vi "item select new.vi"(8 "error in (no error)":errorcluster, 10 "Selection (none)":bool[](array[boolean]), 11 "Listbox or Tree":refnum<vi>) -> (0 "error out":errorcluster, 3 "Ref":refnum<vi>)   [LabVIEW 2020, in "UI_ItemSelect_OpenSource.lvlib"]
doc: "This method will register and initialize the input control reference for usage with this library.\n\nAll cache data is stored in a FGV keyed to the control reference. This means that the user\ndoes not have to pass around any data cache to use this library.\n\nImportant rules:\n- If you edit ItemNames/Tags, then you must call this method to re-initialize the internal cache\n- You can safely call this method twice with a control reference without closing inbetween calls."
uses:
  UI_ItemSelect_OpenSource.lvlib
  SubVIs/item select action.ctl
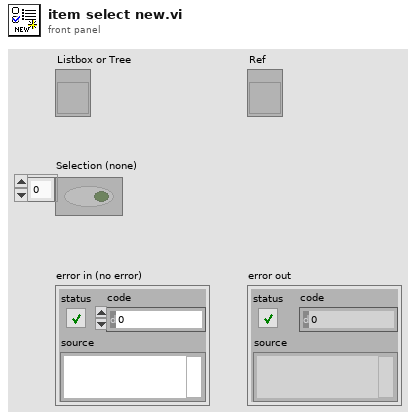
[diagram p1: front panel]
types:
  T1 = typedef "UI_ItemSelect_OpenSource.lvlib/item select action.ctl" = enum16{"init", "read", "write states", "write locks", "mouse down", "delete", "select all", "select none", "invert selection"}
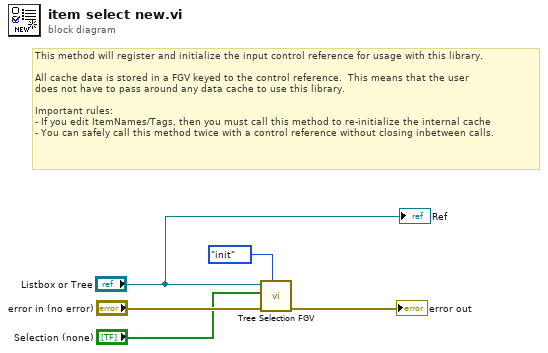
[diagram p0: block diagram]
diagram:
  # "This method will register and initialize the input control reference for usage with this library.\n\nAll cache data is stored in a FGV keyed to the control reference.  This means that the user\ndoes not have to pass around any data cache to use this library.\n\nImportant rules:\n- If you edit ItemNames/Tags, then you must call this method to re-initialize the internal cache\n- You can safely call this method twice with a control reference without closing inbetween calls."
  n1 = call "Tree Selection FGV.vi"("Action"=item_select_action."init", "error in (no error)"="error in (no error)", "States"="Selection (none)", "Listbox or Tree"="Listbox or Tree") -> ("error out"=→"error out":errorcluster)  [unwired: 6 in, 1 out]
  "Ref" <- "Listbox or Tree"
